vi "GA Set Gear Ratio.vi"(6 "lStopSmoothTime":i32, 7 "masterSlope":i32, 8 "error in (no error)":errorcluster caption="错误输入（无错误）", 9 "slaveEven":i32, 10 "masterEven":i32, 11 "nAxisNum":i16) -> (0 "error out":errorcluster caption="错误输出", 3 "function return":i32)   [LabVIEW 2015, in "GAS.lvlib"]
doc: "extern \"C\" __declspec(dllimport) int GA_SetGearRatio(short nAxisNum,long masterEven,long slaveEven,long masterSlope=0,long lStopSmoothTime = 200);"
uses:
  <userlib>/BP_GAS/GAS.lvlib
  <userlib>/BP_GAS/GAS.dll
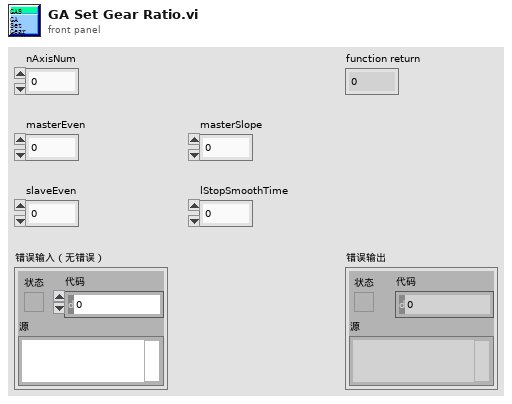
[diagram p1: front panel]
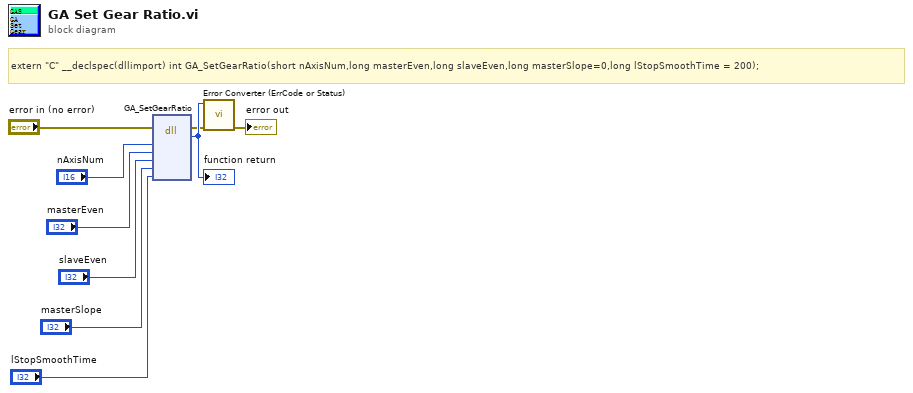
[diagram p0: block diagram]
diagram:
  # "extern \"C\" __declspec(dllimport) int GA_SetGearRatio(short nAxisNum,long masterEven,long slaveEven,long masterSlope=0,long lStopSmoothTime = 200);"
  n1 = dll-call lib="E:/Program Files (x86)/National Instruments/LabVIEW 2015/user.lib/BP_GAS/GAS.*" fn="GA_SetGearRatio"(error in="error in (no error)", "nAxisNum"="nAxisNum", "masterEven"="masterEven", "slaveEven"="slaveEven", "masterSlope"="masterSlope", "lStopSmoothTime"="lStopSmoothTime") -> (error out=w2:errorcluster, w9:i32)  [unwired: 7 in, 1 out]
  "function return" <- w9
  n2 = call "Error Converter (ErrCode or Status).vi"("error in (no error)"=w2, "error code"=w9) -> ("error out"=→"error out":errorcluster)  [unwired: 9 in]
